vi "TCPSettings_Global.vi"() -> ()   [LabVIEW 2018]
panel:
  in  "TCP Settings":cluster{"service name":string, "port":u16}={"service name"="localhost", "port"=6969}
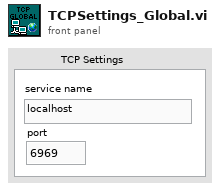
[diagram p1: front panel]
diagram:
